vi "Pylab.vi"() -> ()   [LabVIEW 2015]
uses:
  lab-docs/labVIEW/acquisition/COL/Globals_angles.vi
  <vilib>/picture/3D Picture Control/Object/Create Object (drawable).vi
  <vilib>/picture/3D Picture Control/Object/Add Object (no reference).vi
  <vilib>/picture/3D Picture Control/Object/Add Object (reference).vi
  <vilib>/picture/3D Picture Control/NI_3D Picture Control.lvlib
panel:
  out "3D Picture":refnum<vi>(3d-picture)
  out "yaw":dbl
  out "pitch":dbl
  out "roll":dbl
  in  "Stop Button":bool
  in  "mode (standard)":T1(ring)=enum."CRLF"
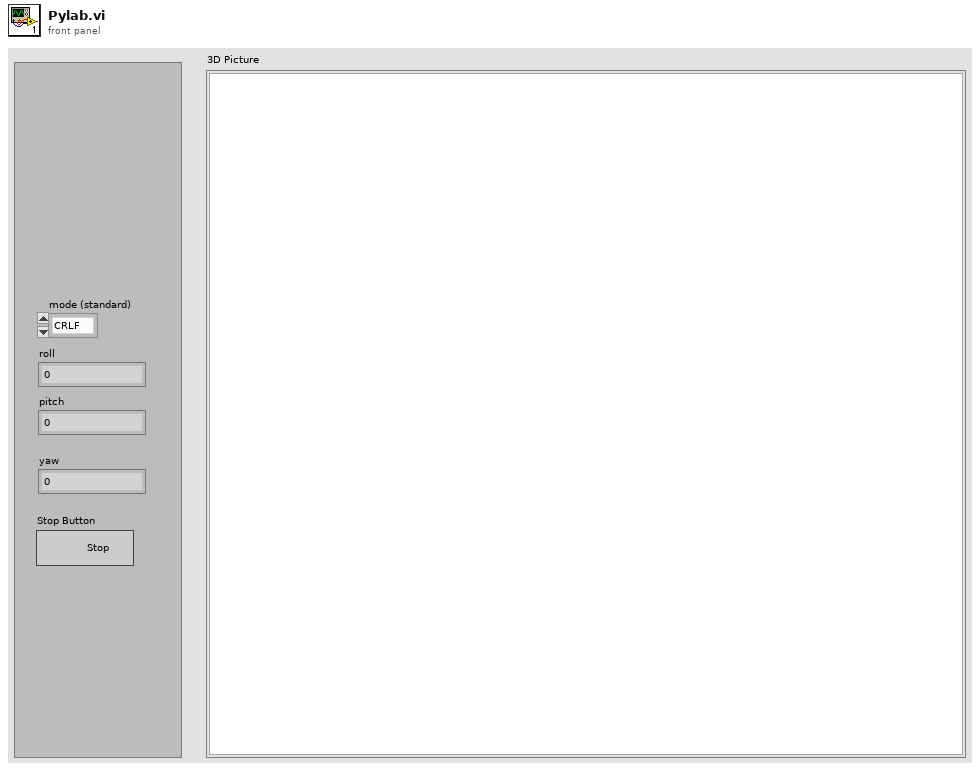
[diagram p1: front panel]
types:
  T1 = enum16{"Standard", "Buffered", "CRLF", "Immediate"}
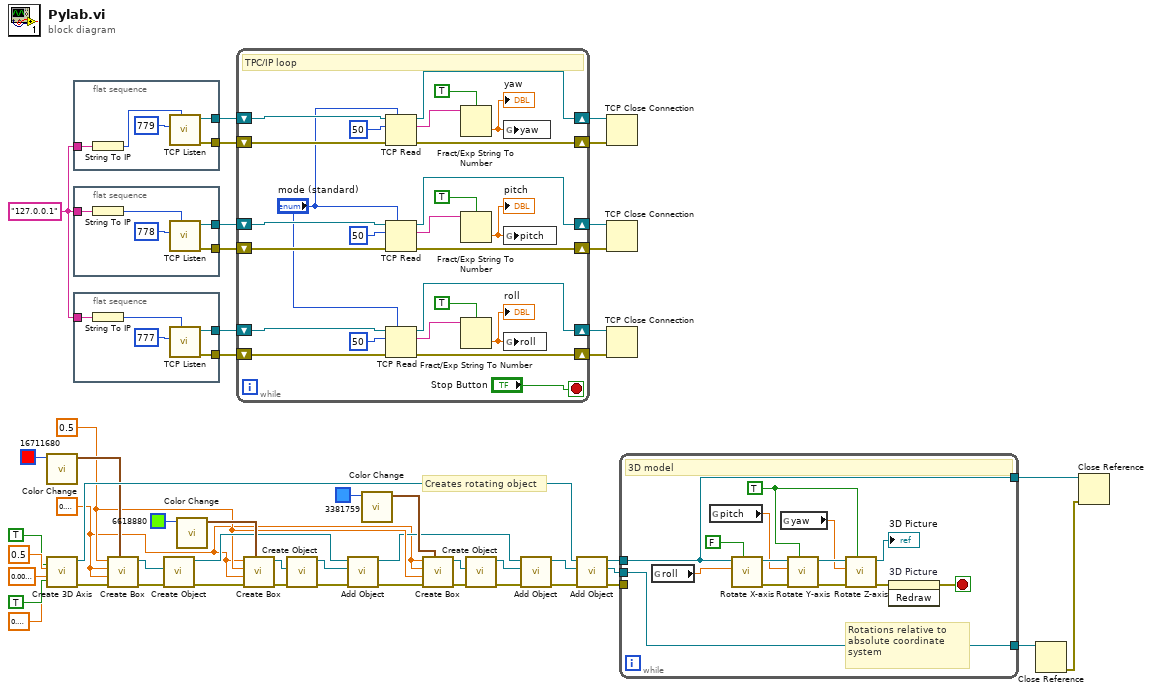
[diagram p0: block diagram]
diagram:
  w7 = sgl 0.1 ("Character Size")
  w16 = sgl 0.5 ("Length")
  w46 = "127.0.0.1"
  # "Creates rotating object"
  n1 = call <vilib>:"Color Change.vi"("Color"=u32 16711680) -> ("RGBA"=w28:cluster{"R":sgl, "G":sgl, "B":sgl, "A":sgl})  [unwired: 10 in]
  n2 = call <vilib>:"Create 3D Axis.vi"("Character Size"=sgl 0.1, "Half plane?"=TRUE, "Axis label?"=TRUE, "Radius"=sgl 0.01, "Length"=sgl 0.5) -> ("error out"=w2:errorcluster, "New Object Refnum"=w32:refnum<vi>)  [unwired: 5 in]
  n3 = flat-sequence {
    tunnel: [w53] -> w38
    tunnel: [w52] -> w39
    tunnel: w46 -> [w51]
    frame #0 {
      n4 = String To IP(1:w51) -> (0:w54:u32)
      n5 = call <vilib>:"TCP Listen.vi"("net address"=w54, "port"=779) -> ("error out"=w53:errorcluster, "connection ID"=w52:refnum<k5>)  [unwired: 5 in, 3 out]
    }
  }
  n6 = flat-sequence {
    tunnel: [w58] -> w44
    tunnel: [w57] -> w45
    tunnel: w46 -> [w56]
    frame #0 {
      n7 = String To IP(1:w56) -> (0:w59:u32)
      n8 = call <vilib>:"TCP Listen.vi"("net address"=w59, "port"=778) -> ("error out"=w58:errorcluster, "connection ID"=w57:refnum<k5>)  [unwired: 5 in, 3 out]
    }
  }
  n9 = flat-sequence {
    tunnel: [w63] -> w50
    tunnel: [w62] -> w49
    tunnel: w46 -> [w61]
    frame #0 {
      n10 = String To IP(1:w61) -> (0:w64:u32)
      n11 = call <vilib>:"TCP Listen.vi"("net address"=w64, "port"=777) -> ("error out"=w63:errorcluster, "connection ID"=w62:refnum<k5>)  [unwired: 5 in, 3 out]
    }
  }
  n12 = call <vilib>:"Create Box.vi"("Color"=w28, "error in (no error)"=w2, "Length Z"=w7, "Length Y"=w7, "Length X"=w16) -> ("error out"=w31:errorcluster, "New Box Refnum"=w30:refnum<vi>)  [unwired: 5 in]
  n13 = call-poly <vilib>:"Create Object.vi"("error in (no error)"=w31, "Geometry"=w30) -> ("error out"=w25:errorcluster, "Scene:New Object"=w22:refnum<vi>)  [unwired: 8 in]
  n14 = call <vilib>:"Color Change.vi"("Color"=u32 6618880) -> ("RGBA"=w23:cluster{"R":sgl, "G":sgl, "B":sgl, "A":sgl})  [unwired: 10 in]
  n15 = while {
    shift-right: [w87] -> w47
    shift-left: w50 -> [w90]
    shift-right: [w88] -> w48
    shift-left: w49 -> [w89]
    shift-right: [w74] -> w42
    shift-left: w44 -> [w76]
    shift-right: [w75] -> w43
    shift-left: w45 -> [w77]
    shift-right: [w73] -> w41
    shift-left: w39 -> [w71]
    shift-right: [w72] -> w40
    shift-left: w38 -> [w70]
    stop <- "Stop Button" stop-if-true
    # "TPC/IP loop"
    n16 = TCP Read(connection ID=w71, bytes to read=50, error in (no error)=w70, 7:"mode (standard)") -> (connection ID out=w73:refnum<k5>, data out=w79:string, error out=w72:errorcluster)  [unwired: 1 in]
    n17 = TCP Read(connection ID=w77, bytes to read=50, error in (no error)=w76, 7:"mode (standard)") -> (connection ID out=w75:refnum<k5>, data out=w82:string, error out=w74:errorcluster)  [unwired: 1 in]
    n18 = TCP Read(connection ID=w89, bytes to read=50, error in (no error)=w90, 7:"mode (standard)") -> (connection ID out=w88:refnum<k5>, data out=w85:string, error out=w87:errorcluster)  [unwired: 1 in]
    n19 = Fract/Exp String To Number(use system decimal point (T)=TRUE, string=w79) -> (number=w67:dbl)  [unwired: 2 in, 1 out]
    "yaw" <- w67
    n20 = Fract/Exp String To Number(use system decimal point (T)=TRUE, string=w82) -> (number=w68:dbl)  [unwired: 2 in, 1 out]
    "pitch" <- w68
    n21 = Fract/Exp String To Number(use system decimal point (T)=TRUE, string=w85) -> (number=w66:dbl)  [unwired: 2 in, 1 out]
    "roll" <- w66
    n22 = global write "Globals_angles.vi" "yaw"(w67) -> ()
    n23 = global write "Globals_angles.vi" "pitch"(w68) -> ()
    n24 = global write "Globals_angles.vi" "roll"(w66) -> ()
  }
  n25 = call <vilib>:"Create Box.vi"("Color"=w23, "error in (no error)"=w25, "Length Z"=w7, "Length Y"=w16, "Length X"=w7) -> ("error out"=w26:errorcluster, "New Box Refnum"=w27:refnum<vi>)  [unwired: 5 in]
  n26 = call-poly <vilib>:"Create Object.vi"("error in (no error)"=w26, "Geometry"=w27) -> ("error out"=w6:errorcluster, "Scene:New Object"=w21:refnum<vi>)  [unwired: 8 in]
  n27 = call-poly <vilib>:"Add Object.vi"("error in (no error)"=w6, "New Object In"=w21, "Scene Object In"=w22) -> ("error out"=w4:errorcluster, "Scene Object Out"=w15:refnum<vi>)  [unwired: 7 in]
  n28 = call <vilib>:"Color Change.vi"("Color"=u32 3381759) -> ("RGBA"=w17:cluster{"R":sgl, "G":sgl, "B":sgl, "A":sgl})  [unwired: 10 in]
  n29 = call <vilib>:"Create Box.vi"("Color"=w17, "error in (no error)"=w4, "Length Z"=w16, "Length Y"=w7, "Length X"=w7) -> ("error out"=w20:errorcluster, "New Box Refnum"=w19:refnum<vi>)  [unwired: 5 in]
  n30 = call-poly <vilib>:"Create Object.vi"("error in (no error)"=w20, "Geometry"=w19) -> ("error out"=w5:errorcluster, "Scene:New Object"=w14:refnum<vi>)  [unwired: 8 in]
  n31 = call-poly <vilib>:"Add Object.vi"("error in (no error)"=w5, "New Object In"=w14, "Scene Object In"=w15) -> ("error out"=w3:errorcluster, "Scene Object Out"=w13:refnum<vi>)  [unwired: 7 in]
  n32 = call-poly <vilib>:"Add Object.vi"("error in (no error)"=w3, "New Object In"=w13, "Scene Object In"=w32) -> ("error out"=w1:errorcluster, "New Object Out"=w11:refnum<vi>, "Scene Object Out"=w12:refnum<vi>)  [unwired: 6 in]
  n33 = TCP Close Connection(connection ID=w41, error in (no error)=w40) -> ()  [unwired: 1 in, 2 out]
  n34 = TCP Close Connection(connection ID=w43, error in (no error)=w42) -> ()  [unwired: 1 in, 2 out]
  n35 = TCP Close Connection(connection ID=w48, error in (no error)=w47) -> ()  [unwired: 1 in, 2 out]
  n36 = while {
    tunnel: w12 -> [w95]
    tunnel: w11 -> [w105]
    tunnel: [w95] -> w10
    tunnel: [w105] -> w9
    tunnel: w1 -> [_]
    stop <- w92 stop-if-true
    w99 = TRUE ("Relative?")
    # "Rotations relative to absolute coordinate system"
    # "3D model"
    n37 = global read "Globals_angles.vi" "roll"() -> (w98:dbl)
    n38 = global read "Globals_angles.vi" "pitch"() -> (w97:dbl)
    n39 = call <vilib>:"Rotate X-axis.vi"("Relative?"=FALSE, "angle"=w98, "Scene Object In"=w95) -> ("error out"=w104:errorcluster, "Scene Object Out"=w103:refnum<vi>)  [unwired: 7 in]
    n40 = global read "Globals_angles.vi" "yaw"() -> (w96:dbl)
    n41 = call <vilib>:"Rotate Y-axis.vi"("Relative?"=w99, "error in (no error)"=w104, "angle"=w97, "Scene Object In"=w103) -> ("error out"=w102:errorcluster, "Scene Object Out"=w101:refnum<vi>)  [unwired: 6 in]
    n42 = call <vilib>:"Rotate Z-axis.vi"("Relative?"=w99, "error in (no error)"=w102, "angle"=w96, "Scene Object In"=w101) -> ("error out"=w93:errorcluster, "Scene Object Out"=→"3D Picture":refnum<vi>)  [unwired: 6 in]
    n43 = invoke on="3D Picture" class="SceneGraphDisp (strict)" method="Redraw"(error in=w93) -> (error out=w92:errorcluster)  [unwired: 2 in, 2 out]
  }
  n44 = Close Reference(reference=w9) -> (error out=w8:errorcluster)  [unwired: 1 in]
  n45 = Close Reference(reference=w10, error in (no error)=w8) -> ()  [unwired: 1 out]
